vi "TCP_Control.vi"() -> ()   [LabVIEW 2013, in "AccelNET.lvlib" / "Control_VIs.lvlib"]
uses:
  <userlib>/Accelerator/Device IO/Pelletron/Accelnet/Control_VIs.lvlib
  <vilib>/Utility/miscctls.llb/LVPointTypeDef.ctl
  <userlib>/Accelerator/Device IO/Pelletron/Accelnet/TCPinfo.vi
  <userlib>/Accelerator/Device IO/Pelletron/Accelnet/TCP.lvclass
  <userlib>/Accelerator/Device IO/Pelletron/Accelnet/Global_Variables.lvlib
panel:
  in  "stop":bool
  in  "Timeout":i32=60000
  in  "Write Port":i16=6181
  in  "Read Port":i16=6180
  in  "Ip Address":string="192.168.1.101"
  out "timeout ms (60000)":i32
  out "Write Port 2":i16
  out "Read Port 2":i16
  out "IP Address":string
  out "Write Error Out":errorcluster
  out "Read Error Out":errorcluster
  in  "Close Connection":bool
  in  "Open Connection":bool
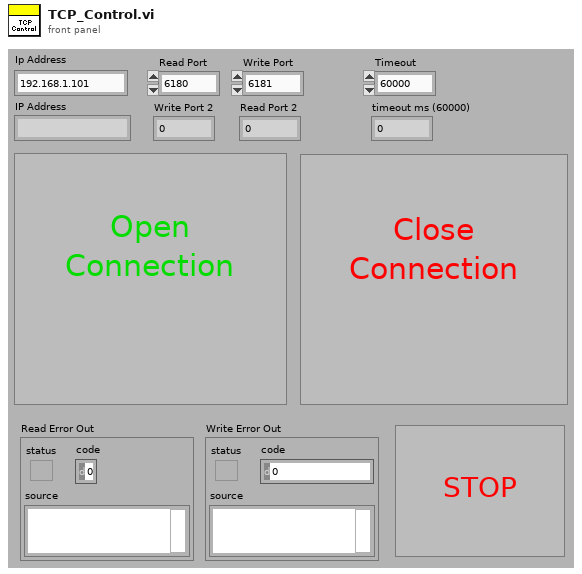
[diagram p1: front panel]
types:
  T1 = typedef "LVPointTypeDef.ctl" = cluster{"Horizontal":i16, "Vertical":i16}
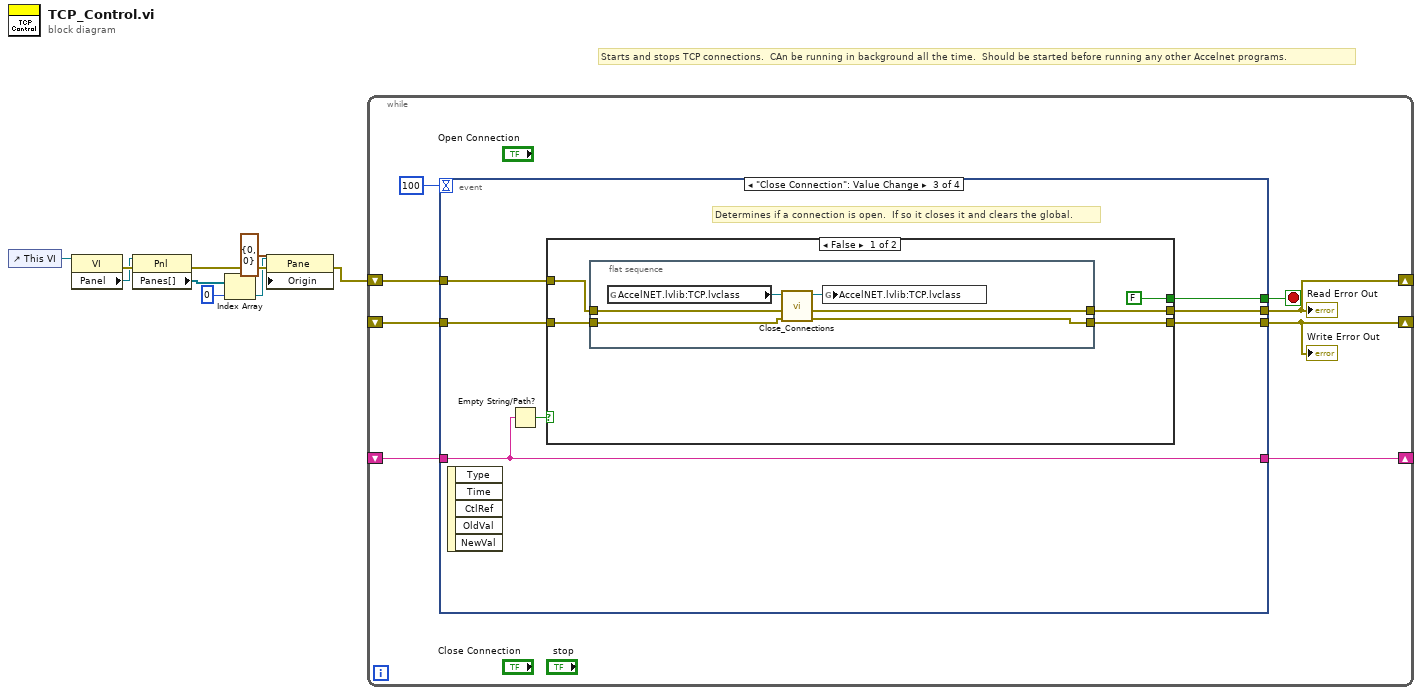
[diagram p0: block diagram]
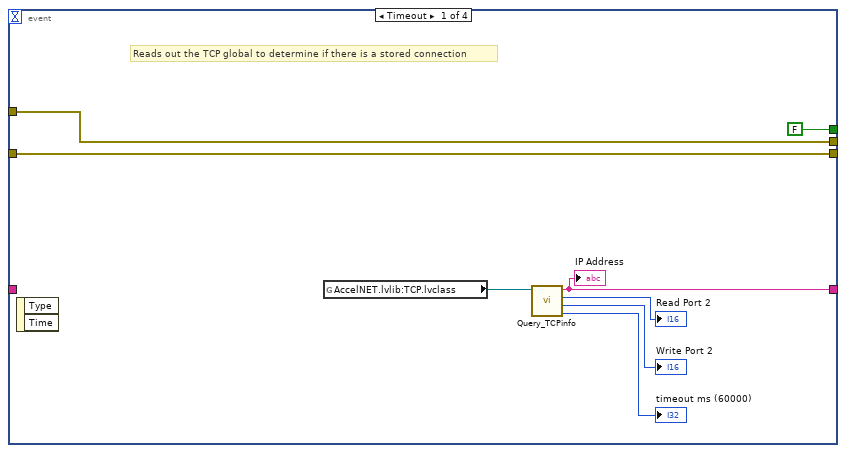
[diagram p2: hidden frame]
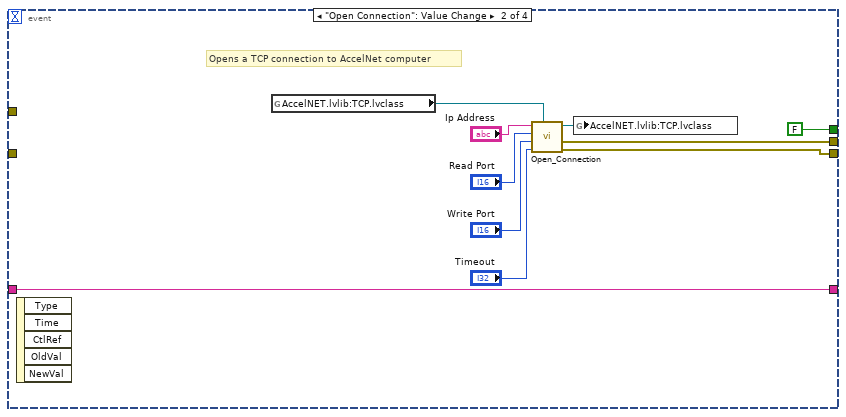
[diagram p3: hidden frame]
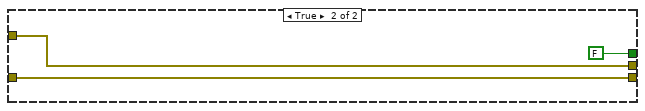
[diagram p4: hidden frame]
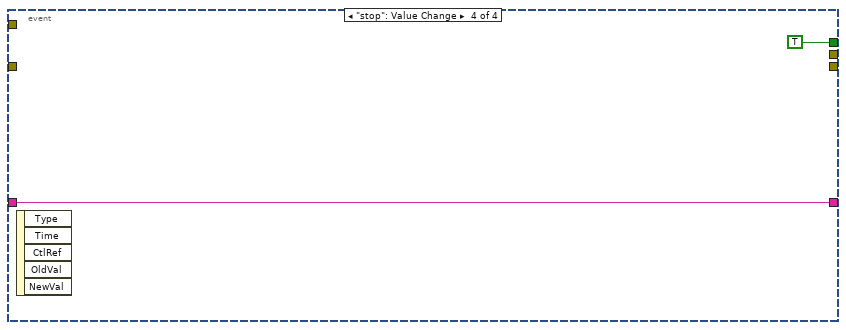
[diagram p5: hidden frame]
diagram:
  # "Starts and stops TCP connections.  CAn be running in background all the time.  Should be started before running any other Accelnet programs."
  n1 = control-ref of="This VI"() -> (w9:refnum<vi>)
  n2 = property class="VI"(reference=w9) -> (error out=w8:errorcluster, "Panel"=w7:refnum<vi>)  [unwired: 1 in, 1 out]
  n3 = property class="Pnl"(reference=w7, error in=w8) -> (error out=w6:errorcluster, "Panes[]"=w5:refnum<vi>[])  [unwired: 1 out]
  n4 = Index Array(array=w5, index=0) -> (element=w3:refnum<vi>)
  n5 = property class="Pane"(reference=w3, error in=w6, "Origin"=T1 {"Horizontal"=0, "Vertical"=0}) -> (error out=w1:errorcluster)  [unwired: 1 out]
  n6 = while {
    shift-right: [w15] -> _
    shift-left: w1 -> [w17]
    shift-right: [w14] -> _
    shift-left: _ -> [w16]
    shift-right: [w12] -> _
    shift-left: _ -> [w11]
    stop <- w13 stop-if-true
    n7 = event shown="[2] \"Close Connection\": Value Change" {
      selector: _ -> [_ _ _ _]
      dyn-events: _ -> [_ _ _ _]
      timeout: 100 -> [_ _ _ _]
      tunnel: [w25 w29 w42 _] -> w15
      tunnel: [w24 w28 w41 _] -> w14
      tunnel: w17 -> [w25 _ w40 _]
      tunnel: w16 -> [w24 _ w39 _]
      tunnel: [FALSE FALSE w38 TRUE] -> w13
      tunnel: [w18 w26 w36 w57] -> w12
      tunnel: w11 -> [_ w26 w36 w57]
      event Timeout {
        # "Reads out the TCP global to determine if there is a stored connection"
        n8 = event-data() -> ()  [unwired: 1 in, 2 out]
        n9 = global read "TCPinfo.vi" "AccelNET.lvlib:TCP.lvclass"() -> (w19:refnum<class "TCP.lvclass">)
        n10 = call <userlib>:"Query_TCPinfo.vi"("AccelNET.lvlib:TCP.lvclass"=w19) -> ("timeout ms (60000)"=→"timeout ms (60000)":i32, "Write Port"=→"Write Port 2":i16, "Read Port"=→"Read Port 2":i16, "IP Address"=w18:string)  [unwired: 5 in, 2 out]
        "IP Address" <- w18
      }
      event "Open Connection": Value Change {
        # "Opens a TCP connection to AccelNet computer"
        n11 = event-data() -> ()  [unwired: 1 in, 5 out]
        n12 = global read "TCPinfo.vi" "AccelNET.lvlib:TCP.lvclass"() -> (w30:refnum<class "TCP.lvclass">)
        n13 = call <userlib>:"Open_Connection.vi"("AccelNET.lvlib:TCP.lvclass"=w30, "timeout ms (60000)"="Timeout", "Write Port"="Write Port", "Read Port"="Read Port", "IP Address"="Ip Address") -> ("Write Error"=w28:errorcluster, "Read Error"=w29:errorcluster, "AccelNET.lvlib:TCP.lvclass 2"=w31:refnum<class "TCP.lvclass">)  [unwired: 2 in, 2 out]
        n14 = global write "TCPinfo.vi" "AccelNET.lvlib:TCP.lvclass"(w31) -> ()
      }
      event "Close Connection": Value Change {
        # "Determines if a connection is open.  If so it closes it and clears the global."
        n15 = event-data() -> ()  [unwired: 1 in, 5 out]
        n16 = Empty String/Path?(string/path=w36) -> (empty?=w37:bool)
        n17 = case shown="False" w37 {
          tunnel: [w47 w55] -> w42
          tunnel: [w46 w56] -> w41
          tunnel: w40 -> [w45 w55]
          tunnel: w39 -> [w44 w56]
          tunnel: [FALSE FALSE] -> w38
          frame False {
            n18 = flat-sequence {
              tunnel: w45 -> [w51]
              tunnel: w44 -> [w50]
              tunnel: [w53] -> w47
              tunnel: [w52] -> w46
              frame #0 {
                n19 = global read "TCPinfo.vi" "AccelNET.lvlib:TCP.lvclass"() -> (w49:refnum<class "TCP.lvclass">)
                n20 = call <userlib>:"Close_Connections.vi"("Write Error in"=w50, "Read Error in"=w51, "AccelNET.lvlib:TCP.lvclass"=w49) -> ("Write Error Out"=w52:errorcluster, "Read Error Out"=w53:errorcluster, "AccelNET.lvlib:TCP.lvclass 2"=w48:refnum<class "TCP.lvclass">)  [unwired: 6 in]
                n21 = global write "TCPinfo.vi" "AccelNET.lvlib:TCP.lvclass"(w48) -> ()
              }
            }
          }
          frame True {
          }
        }
      }
      event "stop": Value Change {
        n22 = event-data() -> ()  [unwired: 1 in, 5 out]
      }
    }
    "Read Error Out" <- w15
    "Write Error Out" <- w14
  }
